vi "same loop.vi"() -> ()   [LabVIEW 2014]
uses:
  <vilib>/LVH/AR Drone Toolkit/Decode NavData/Typedefs/NavData Demo.ctl
  <vilib>/LVH/AR Drone Toolkit/AR Drone.lvlib
panel:
  in  "NavData Out":T1
  out "NavData Out 2":T1
  in  "Setup Parameters":T2={"Drone IP address"="192.168.1.1", "Home IP address"="192.168.1.2", "Flight Mode"=enum."INDOOR MODE", "Mounted Hull"=enum."INDOOR HULL", "Video Camera"=2, "Max Altitude (m)"=3.0, "Max Pitch and Roll Angle (deg)"=10.0, "Max Vertical Speed (m/s)"=0.7, "Max Yaw Speed (deg/s)"=100.0} {"Video Camera" items=["Bottom Camera"=1, "Front Camera"=0, "Front in Bottom"=3, "Bottom in Front"=2]}
  out "Control cluster":T3 {"Roll" scale=-1.0..1.0; "Pitch" scale=-1.0..1.0; "Vertical Speed" scale=-1.0..1.0; "Yaw Speed" scale=-1.0..1.0}
  out "Video Stream":picture
  in  "Emergency Landing":bool
  in  "Takeoff/Land":bool
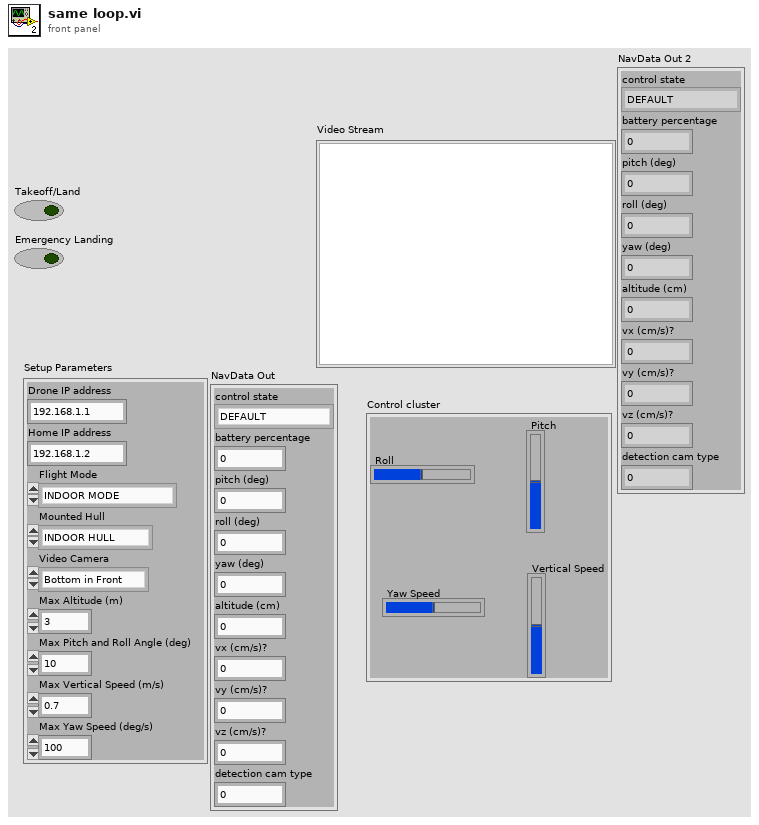
[diagram p1: front panel]
types:
  T1 = typedef "AR Drone.lvlib/NavData Demo.ctl" = cluster{"control state":enum32{"DEFAULT", "INIT", "LANDING", "FLYING", "HOVERING", "TEST", "TRANS_TAKEOFF", "TRANS_GOTOFIX", "TRANS_LANDING"}, "battery percentage":u32, "pitch (deg)":sgl, "roll (deg)":sgl, "yaw (deg)":sgl, "altitude (cm)":u32, "vx (cm/s)?":sgl, "vy (cm/s)?":sgl, "vz (cm/s)?":sgl, "detection cam type":u32}
  T2 = cluster{"Drone IP address":string, "Home IP address":string, "Flight Mode":enum8{"OUTDOOR MODE", "INDOOR MODE"}, "Mounted Hull":enum8{"OUTDOOR HULL", "INDOOR HULL"}, "Video Camera":u8, "Max Altitude (m)":sgl, "Max Pitch and Roll Angle (deg)":sgl, "Max Vertical Speed (m/s)":sgl, "Max Yaw Speed (deg/s)":sgl}
  T3 = cluster{"Roll":dbl, "Pitch":dbl, "Vertical Speed":dbl, "Yaw Speed":dbl}
  T4 = typedef "AR Drone.lvlib/AR Drone Resource.ctl" = cluster{"UDP Control Connection":refnum<k16>, "UDP NavData Connection":refnum<k16>, "UDP Video Connection (Drone 1.0)":refnum<k16>, "TCP Video Connection (Drone 2.0)":refnum<k5>, "TCP Control Port Connection":refnum<k5>, "Drone IP address":string, "Drone Command Port":u16, "Drone NavData Port":u16, "Drone Vid Stream Port":u16, "Drone TCP Control Port":u16, "Home IP address":string, "Home Command Port":u16, "Home NavData Port":u16, "Home Vid Stream Port":u16, "Drone Version":i32, "Drone Index":i32, "Command Sequence":i32}
  T5 = cluster{"Hover":bool, bool, "Emergency Landing":bool, "button 4":bool, "button 5":bool, "button 6":bool, "button 7":bool, "button 8":bool}
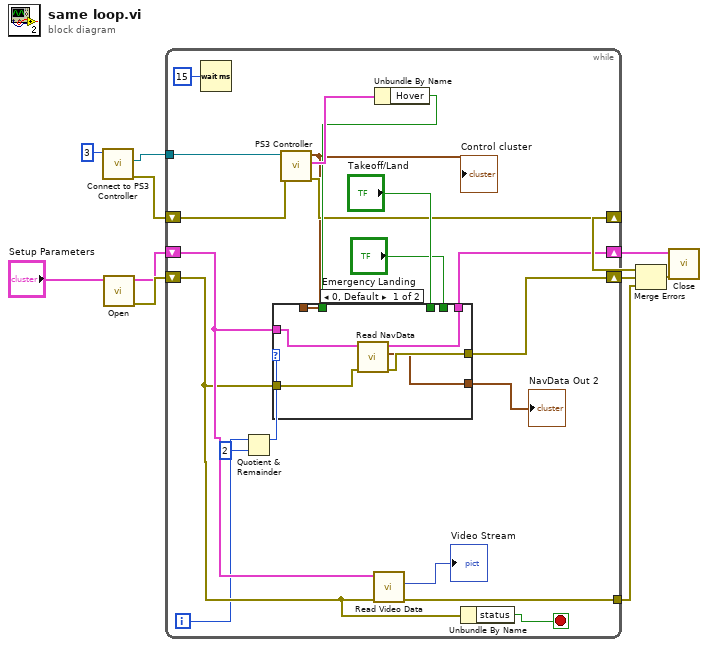
[diagram p0: block diagram]
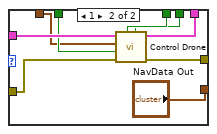
[diagram p2: hidden frame]
diagram:
  n1 = call "Connect to PS3 Controller.vi"("device ID"=3) -> ("error out"=w11:errorcluster, "device ID 2"=w10:refnum<k1>)  [unwired: 7 in, 1 out]
  n2 = call <vilib>:"Open.vi"("Setup Parameters"="Setup Parameters") -> ("error out"=w8:errorcluster, "AR Drone Resource"=w7:T4)  [unwired: 9 in]
  n3 = while {
    tunnel: w10 -> [w30]
    tunnel: [w20] -> w1
    shift-right: [w23] -> w4
    shift-left: w11 -> [w31]
    shift-right: [w22] -> w3
    shift-left: w8 -> [w16]
    shift-right: [w24] -> w6
    shift-left: w7 -> [w29]
    i -> [w14]
    stop <- w19 stop-if-true
    n4 = Wait (ms)(milliseconds to wait=u32 15) -> ()  [unwired: 1 out]
    n5 = Quotient & Remainder(x=w14, y=2) -> (x-y*floor(x/y)=w12:i32)  [unwired: 1 out]
    n6 = call "PS3 Controller.vi"("error in (no error)"=w31, "device ID"=w30) -> ("error out"=w23:errorcluster, "Buttons"=w26:T5, "Control cluster"=w18:T3)  [unwired: 6 in, 1 out]
    "Control cluster" <- w18
    n7 = call <vilib>:"Read Video Data.vi"("error in (no error)"=w16, "AR Drone Resource"=w29) -> ("error out"=w20:errorcluster, "Video Stream"=→"Video Stream":picture)  [unwired: 7 in, 1 out]
    n8 = Unbundle By Name(w26) -> ("Hover"=w25:bool)
    n9 = case shown="0, Default" w12 {
      tunnel: w29 -> [w36 w45]
      tunnel: "Takeoff/Land" -> [_ w44]
      tunnel: "Emergency Landing" -> [_ w43]
      tunnel: w25 -> [_ w42]
      tunnel: [w32 w41] -> w24
      tunnel: [w35 w40] -> w22
      tunnel: w18 -> [_ w39]
      tunnel: w16 -> [w34 w38]
      tunnel: [w33 "NavData Out"] -> w15
      frame 0, Default {
        n10 = call <vilib>:"Read NavData.vi"("error in (no error)"=w34, "AR Drone Resource"=w36) -> ("error out"=w35:errorcluster, "NavData Out"=w33:T1, "AR Drone Resource Out"=w32:T4)  [unwired: 7 in]
      }
      frame 1 {
        n11 = call <vilib>:"Control Drone.vi"("Emergency Landing"=w43, "Takeoff/Land"=w44, "error in (no error)"=w38, "Hover"=w42, "Control Cluster"=w39, "AR Drone Resource"=w45) -> ("error out"=w40:errorcluster, "AR Drone Resource Out"=w41:T4)  [unwired: 4 in]
      }
    }
    "NavData Out 2" <- w15
    n12 = Unbundle By Name(w16) -> ("status"=w19:bool)
  }
  n13 = Merge Errors(w4, w3, w1) -> (w5:errorcluster)
  n14 = call <vilib>:"Close.vi"("error in (no error)"=w5, "AR Drone Resource"=w6) -> ()  [unwired: 9 in, 1 out]
